vi "Actor Core.vi"(8 "error in":errorcluster, 11 "CameraTestingUI in":refnum<class "CameraTestingUI.lvclass">) -> (0 "error out":errorcluster, 3 "Actor out":refnum<class "Actor.lvclass">)   [LabVIEW 2020, in "CameraTestingUI.lvlib" / "CameraTestingUI.lvclass"]
doc: "(<B>Filename</B>: Actor Framework.lvlib:Actor.lvclass:Actor Core.vi)\n\nReceives messages to the actor, reacts to them, and initiates any error handling that may shut the actor down.\n\nDescendant classes may override this VI to append parallel tasks for the actor to complete while it handles messages. Overrides use the Call Parent Class Method node."
uses:
  CameraTestingUI.lvclass
  C:/Program Files (x86)/National Instruments/LabVIEW 2020/vi.lib/ActorFramework/Actor/Actor.lvclass
  <vilib>/ActorFramework/Actor/Actor.lvclass
  Private/TypeDef/ConnectCamera.ctl
  Private/TypeDef/DisconnectCamera.ctl
  Private/TypeDef/CommandParameters.ctl
  Private/TypeDef/SetParams.ctl
  Private/TypeDef/GetParams.ctl
  Private/TypeDef/SnapShot.ctl
  Private/TypeDef/StartStreamVideo.ctl
  Private/TypeDef/StopStreamVideo.ctl
  Private/TypeDef/Quit.ctl
  Private/TypeDef/ViewerTab.ctl
  Private/TypeDef/ConnectionStatus.ctl
  CameraTestingUI.lvclass/CameraTestingUI.ctl
  <vilib>/ActorFramework/Actor/Actor.lvclass/Actor.ctl
  <vilib>/ActorFramework/Message Enqueuer/Message Enqueuer.lvclass/Message Enqueuer.ctl
  Private/TypeDef/VideoLoopCamTestEvn.ctl
  ICameraTesting/ICameraTesting/TypeDef/VideoBufferUpdate.ctl
  <vilib>/picture/picture.llb/imagedata.ctl
  Private/TypeDef/HelperLoopCamTestEvn.ctl
  Camera/ICamera/ICamera/TypeDef/SnapInfo.ctl
  ICameraTesting/ICameraTesting/TypeDef/FrameRateValReceived.ctl
  ICameraTesting/ICameraTesting/TypeDef/ImgTypeValReceived.ctl
  ICameraTesting/ICameraTesting/TypeDef/ResolutionValReceived.ctl
  ICameraTesting/ICameraTesting/TypeDef/VideoOptCodesUpdated.ctl
  ICameraTesting/ICameraTesting/TypeDef/VideoOptionsInfo.ctl
  ICameraTesting/ICameraTesting/TypeDef/StatusUpdated.ctl
  ICameraTesting/ICameraTesting/TypeDef/StatusRecord.ctl
  CameraTestingUI Messages/onVideoOptInfoUpd Msg/onVideoOptInfoUpd Msg.lvclass/onVideoOptInfoUpd Msg.ctl
  CameraTestingUI Messages/onStatusUpdated Msg/onStatusUpdated Msg.lvclass/onStatusUpdated Msg.ctl
  ICameraTesting/ICameraTesting Messages/SetImageType Msg/SetImageType Msg.lvclass/SetImageType Msg.ctl
  ICameraTesting/ICameraTesting Messages/SetResolution Msg/SetResolution Msg.lvclass/SetResolution Msg.ctl
  ICameraTesting/ICameraTesting Messages/SetFrameRate Msg/SetFrameRate Msg.lvclass/SetFrameRate Msg.ctl
  <vilib>/ActorFramework/Message Enqueuer/Init from Existing Queue.vi
  <vilib>/ActorFramework/Message Enqueuer/Enqueue.vi
  CameraTestingUI Messages/onVideoOptInfoUpd Msg/onVideoOptInfoUpd Msg.lvclass
  C:/Program Files (x86)/National Instruments/LabVIEW 2020/vi.lib/ActorFramework/Message/Message.lvclass
  CameraTestingUI Messages/onStatusUpdated Msg/onStatusUpdated Msg.lvclass
  ICameraTesting/ICameraTesting Messages/ConnectCamera Msg/ConnectCamera Msg.lvclass
  ICameraTesting/ICameraTesting Messages/DisconnectCamera Msg/DisconnectCamera Msg.lvclass
  ICameraTesting/ICameraTesting Messages/SetImageType Msg/SetImageType Msg.lvclass
  ICameraTesting/ICameraTesting Messages/SetResolution Msg/SetResolution Msg.lvclass
  ICameraTesting/ICameraTesting Messages/SetFrameRate Msg/SetFrameRate Msg.lvclass
  ICameraTesting/ICameraTesting Messages/GetImageType Msg/GetImageType Msg.lvclass
  ICameraTesting/ICameraTesting Messages/GetResolution Msg/GetResolution Msg.lvclass
  ICameraTesting/ICameraTesting Messages/GetFrameRate Msg/GetFrameRate Msg.lvclass
  ICameraTesting/ICameraTesting Messages/SingleShot Msg/SingleShot Msg.lvclass
  ICameraTesting/ICameraTesting Messages/StartStreaming Msg/StartPlay Msg.lvclass
  ICameraTesting/ICameraTesting Messages/StopStreaming Msg/StopPlayMsg.lvclass
  <vilib>/ActorFramework/Stop Msg/Stop Msg.lvclass
  <vilib>/ActorFramework/Message Priority Queue/Priority Enqueue.vi
  <vilib>/ActorFramework/Message Enqueuer/Message Enqueuer.lvclass
  E:/GitHub/Evaluation_Test/Labview/src/CameraTestingApp/CameraTestingUI/CameraTestingUI/CameraTestingUI.lvclass
  E:/GitHub/Evaluation_Test/Labview/src/CameraTestingApp/ICameraTestingUI/ICameraTestingUI/ICameraTestingUI.lvclass
  ICameraTesting/ICameraTesting/ICameraTesting.lvclass
  Camera/ICamera/ICamera/ICamera.lvclass
panel:
  in  "ViewerTab":T1 caption="Viewer"
  out "ImgViewer":picture
  out "StatusLog":string caption="Status Log"
  in  "StopVideo":T2 caption="Stop"
  in  "PlayVideo":T3 caption="Play"
  in  "OneShot":T4 caption="SnapShot"
  in  "SetParam":T5 caption="Set Parameter"
  in  "GetParam":T6 caption="Get Paramameter"
  in  "CommParams":T7 caption="Command Parameters"
  out "ImgTypeInd":string caption="Last Value"
  in  "ImgTypeSlct":u8(ring) caption="List"
  out "ResolutionInd":string caption="Last Value"
  in  "ResSlct":u8(ring) caption="List"
  out "FrameRateInd":string caption="Last Value"
  in  "FrameRateSlct":u8(ring) caption="List"
  out "CameraLink":T8 caption="Connection status" items=["Disconnected", "Connected", "Error"]
  in  "Quit":T9
  in  "DisconnectCamera":T10 caption="Disconnect Camera"
  in  "ConnectCamera":T11 caption="Connect Camera"
  # "Parameters"
  # "Actions"
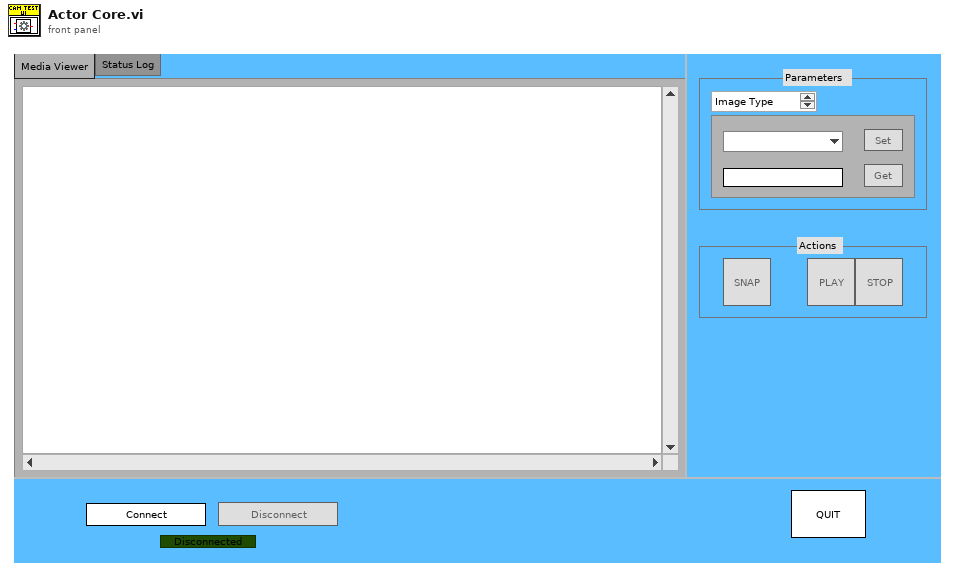
[diagram p1: front panel]
types:
  T1 = typedef "CameraTestingUI.lvlib/CameraTestingUI.lvclass/ViewerTab.ctl" = enum32{"Media Viewer", "Status Log"}
  T2 = typedef "CameraTestingUI.lvlib/CameraTestingUI.lvclass/StopStreamVideo.ctl" = bool
  T3 = typedef "CameraTestingUI.lvlib/CameraTestingUI.lvclass/StartStreamVideo.ctl" = bool
  T4 = typedef "CameraTestingUI.lvlib/CameraTestingUI.lvclass/SnapShot.ctl" = bool
  T5 = typedef "CameraTestingUI.lvlib/CameraTestingUI.lvclass/SetParams.ctl" = bool
  T6 = typedef "CameraTestingUI.lvlib/CameraTestingUI.lvclass/GetParams.ctl" = bool
  T7 = typedef "CameraTestingUI.lvlib/CameraTestingUI.lvclass/CommandParameters.ctl" = enum32{"Image Type", "Resolution", "Frame Rate"}
  T8 = typedef "CameraTestingUI.lvlib/CameraTestingUI.lvclass/ConnectionStatus.ctl" = u16
  T9 = typedef "CameraTestingUI.lvlib/CameraTestingUI.lvclass/Quit.ctl" = bool
  T10 = typedef "CameraTestingUI.lvlib/CameraTestingUI.lvclass/DisconnectCamera.ctl" = bool
  T11 = typedef "CameraTestingUI.lvlib/CameraTestingUI.lvclass/ConnectCamera.ctl" = bool
  T12 = typedef "CameraTestingUI.lvlib/CameraTestingUI.lvclass/HelperLoopEvntRegRef.ctl" = refnum<event-registration>
  T13 = typedef "CameraTestingUI.lvlib/CameraTestingUI.lvclass/VideoLoopEnvRgstRef.ctl" = refnum<event-registration>
  T14 = typedef "CameraTestingUI.lvlib/CameraTestingUI.lvclass/HelperLoopCamTestEvn.ctl" = cluster{"NewSnapData":refnum<user-event>, "FrameRateValReceived":T15, "ImgTypeValReceived":T16, "ResolutionValReceived":T17, "VideoOptInfoUpdated":T18, "StatusUpdated":T19}
  T15 = typedef "ICameraTesting.lvlib/ICameraTesting.lvclass/FrameRateValReceived.ctl" = refnum<user-event>
  T16 = typedef "ICameraTesting.lvlib/ICameraTesting.lvclass/ImgTypeValReceived.ctl" = refnum<user-event>
  T17 = typedef "ICameraTesting.lvlib/ICameraTesting.lvclass/ResolutionValReceived.ctl" = refnum<user-event>
  T18 = typedef "ICameraTesting.lvlib/ICameraTesting.lvclass/VideoOptCodesUpdated.ctl" = refnum<user-event>
  T19 = typedef "ICameraTesting.lvlib/ICameraTesting.lvclass/StatusUpdated.ctl" = refnum<user-event>
  T20 = typedef "imagedata.ctl" = cluster{"image type":i32, "image depth":i32, "image":u8[], "mask":u8[], "colors":u32[], "Rectangle":cluster{"left":i16, "top":i16, "right":i16, "bottom":i16}}
  T21 = typedef "ICameraTesting.lvlib/ICameraTesting.lvclass/VideoOptionsInfo.ctl" = cluster{"FrameRateCodesList":cluster{"Description":string, "Code":u8}[], "VideoResolutionCodesList":cluster{"Description":string, "Code":u8}[], "ImageTypeCodesList":cluster{"Description":string, "Code":u8}[]}
  T22 = typedef "ICameraTesting.lvlib/ICameraTesting.lvclass/StatusRecord.ctl" = cluster{"Time Stamp":timestamp, "Text":string, "Error":errorcluster}
  T23 = typedef "CameraTestingUI.lvlib/CameraTestingUI.lvclass/VideoLoopCamTestEvn.ctl" = cluster{"VideoBufferUpdate":T24}
  T24 = typedef "ICameraTesting.lvlib/ICameraTesting.lvclass/VideoBufferUpdate.ctl" = refnum<user-event>
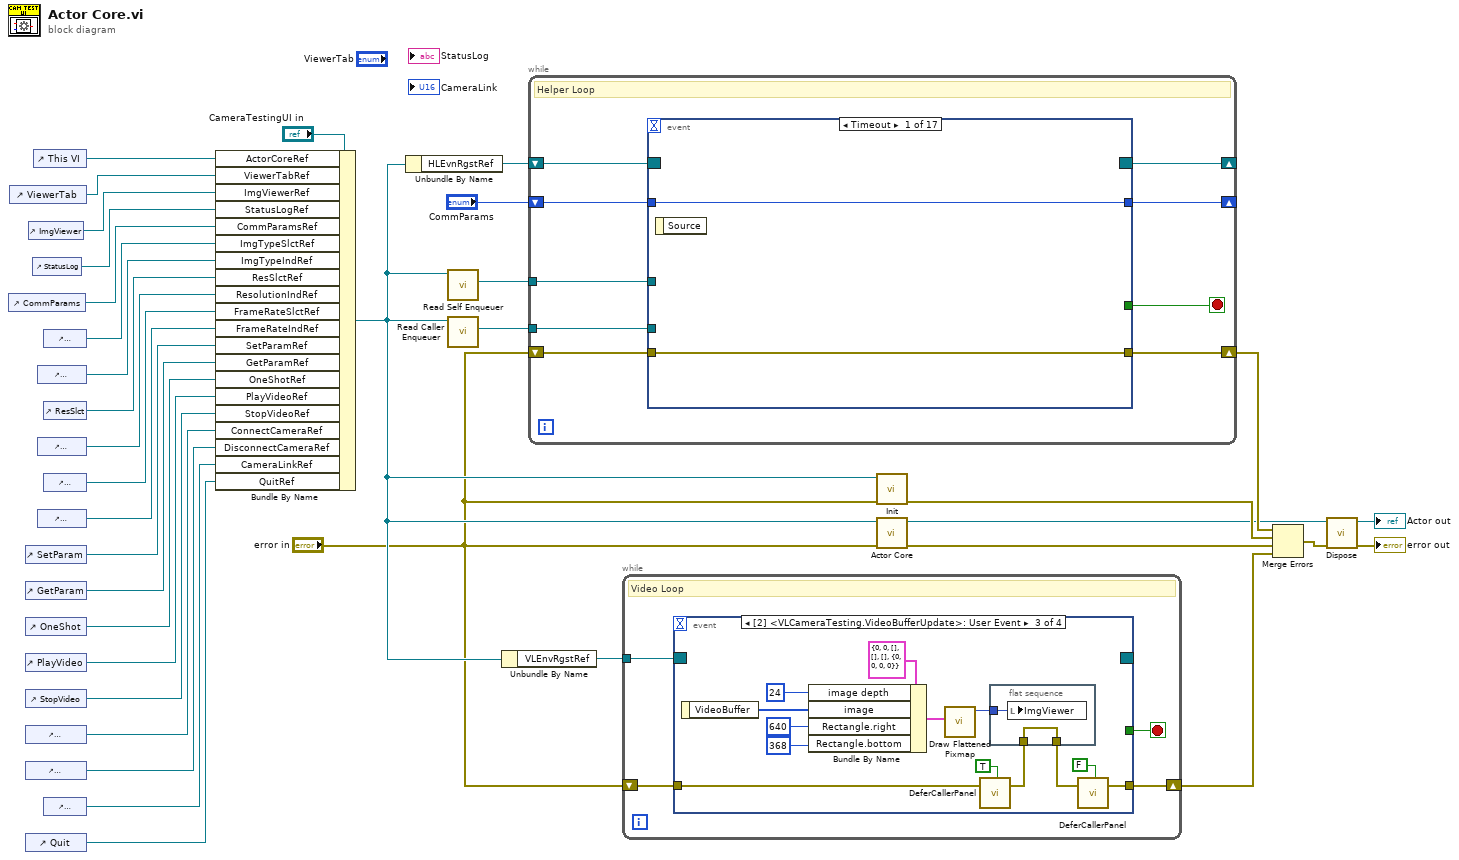
[diagram p0: block diagram]
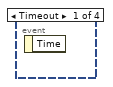
[diagram p2: hidden frame]
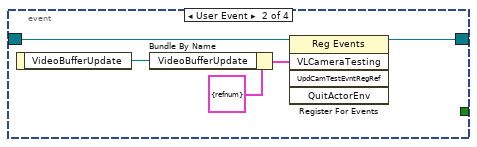
[diagram p3: hidden frame]
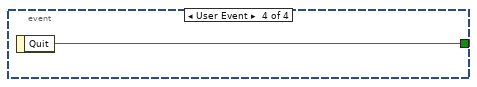
[diagram p4: hidden frame]
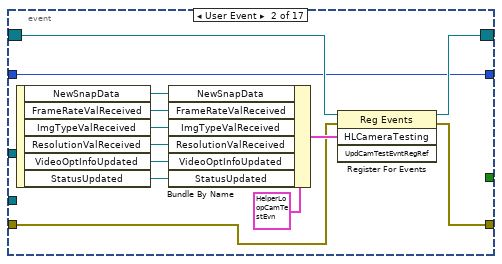
[diagram p5: hidden frame]
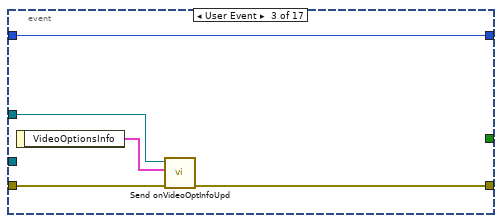
[diagram p6: hidden frame]
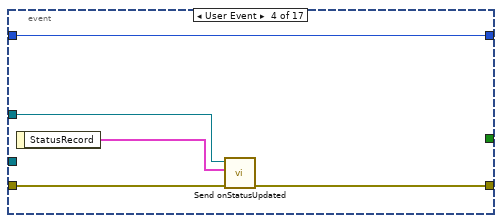
[diagram p7: hidden frame]
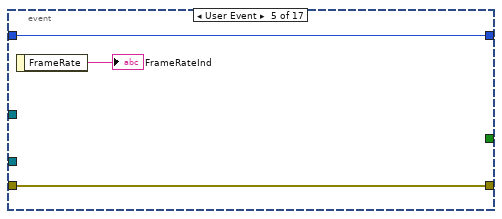
[diagram p8: hidden frame]
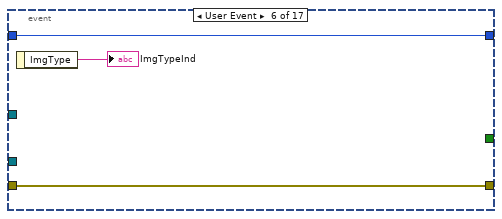
[diagram p9: hidden frame]
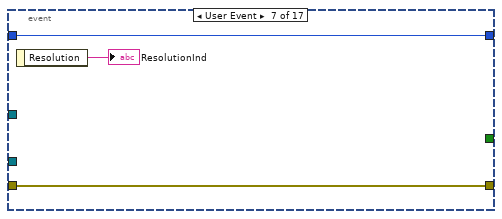
[diagram p10: hidden frame]
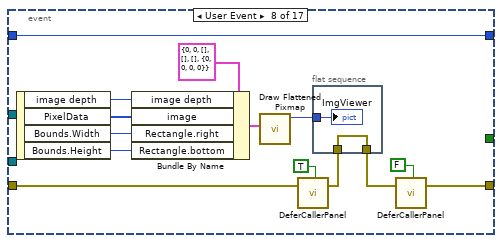
[diagram p11: hidden frame]
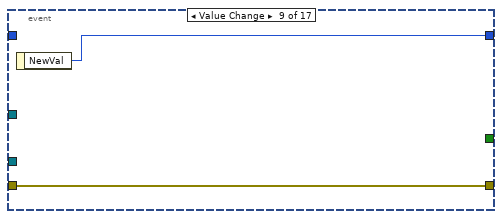
[diagram p12: hidden frame]
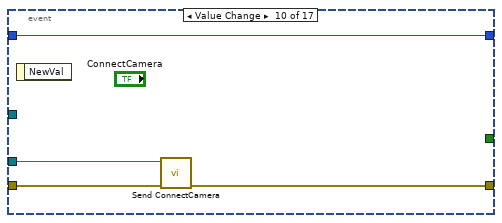
[diagram p13: hidden frame]
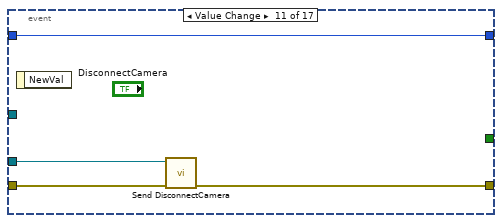
[diagram p14: hidden frame]
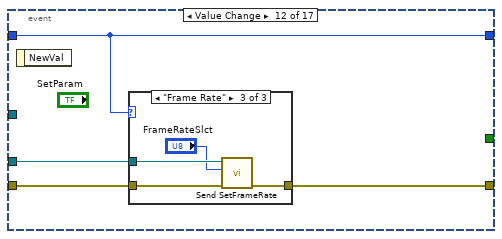
[diagram p15: hidden frame]
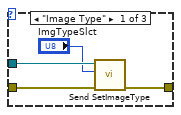
[diagram p16: hidden frame]
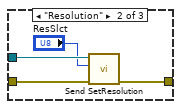
[diagram p17: hidden frame]
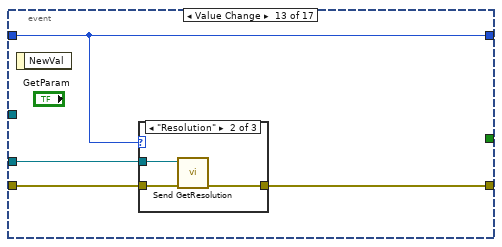
[diagram p18: hidden frame]
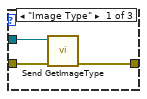
[diagram p19: hidden frame]
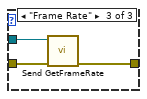
[diagram p20: hidden frame]
diagram:
  n1 = control-ref of="CommParams"() -> (w29:refnum<vi>)
  n2 = control-ref of="ViewerTab"() -> (w32:refnum<vi>)
  n3 = control-ref of="SetParam"() -> (w21:refnum<vi>)
  n4 = control-ref of="GetParam"() -> (w20:refnum<vi>)
  n5 = control-ref of="OneShot"() -> (w19:refnum<vi>)
  n6 = control-ref of="PlayVideo"() -> (w18:refnum<vi>)
  n7 = control-ref of="StopVideo"() -> (w17:refnum<vi>)
  n8 = control-ref of="ConnectCamera"() -> (w16:refnum<vi>)
  n9 = control-ref of="DisconnectCamera"() -> (w15:refnum<vi>)
  n10 = control-ref of="Quit"() -> (w11:refnum<vi>)
  n11 = control-ref of="ImgViewer"() -> (w31:refnum<vi>)
  n12 = control-ref of="StatusLog"() -> (w30:refnum<vi>)
  n13 = control-ref of="This VI"() -> (w34:refnum<vi>)
  n14 = control-ref of="ImgTypeInd"() -> (w27:refnum<vi>)
  n15 = control-ref of="ResolutionInd"() -> (w24:refnum<vi>)
  n16 = control-ref of="FrameRateInd"() -> (w22:refnum<vi>)
  n17 = control-ref of="ImgTypeSlct"() -> (w28:refnum<vi>)
  n18 = control-ref of="ResSlct"() -> (w25:refnum<vi>)
  n19 = control-ref of="FrameRateSlct"() -> (w23:refnum<vi>)
  n20 = control-ref of="CameraLink"() -> (w14:refnum<vi>)
  n21 = Bundle By Name(cluster="CameraTestingUI in", "ActorCoreRef"=w34, "ViewerTabRef"=w32, "ImgViewerRef"=w31, "StatusLogRef"=w30, "CommParamsRef"=w29, "ImgTypeSlctRef"=w28, "ImgTypeIndRef"=w27, "ResSlctRef"=w25, "ResolutionIndRef"=w24, "FrameRateSlctRef"=w23, "FrameRateIndRef"=w22, "SetParamRef"=w21, "GetParamRef"=w20, "OneShotRef"=w19, "PlayVideoRef"=w18, "StopVideoRef"=w17, "ConnectCameraRef"=w16, "DisconnectCameraRef"=w15, "CameraLinkRef"=w14, "QuitRef"=w11) -> (w12:refnum<class "CameraTestingUI.lvclass">)
  n22 = Unbundle By Name(w12) -> ("HLEvnRgstRef"=w33:T12)
  n23 = call <vilib>:"Read Self Enqueuer.vi"("Actor"=w12) -> ("Self Enqueuer"=w13:refnum<class "Message Enqueuer.lvclass">)  [unwired: 10 in]
  n24 = call <vilib>:"Read Caller Enqueuer.vi"("Actor"=w12) -> ("Caller Enqueuer"=w35:refnum<class "Message Enqueuer.lvclass">)  [unwired: 10 in]
  n25 = Unbundle By Name(w12) -> ("VLEnvRgstRef"=w10:T13)
  n26 = while {
    tunnel: w35 -> [w45]
    shift-right: [w43] -> _
    shift-left: "CommParams" -> [w44]
    shift-right: [w40] -> _
    shift-left: w33 -> [w41]
    tunnel: w13 -> [w39]
    shift-right: [w38] -> w8
    shift-left: "error in" -> [w37]
    stop <- w42 stop-if-true
    # "Helper Loop"
    n27 = event shown="[0] Timeout" {
      selector: w41 -> [_ w60 _ _ _ _ _ _ _ _ _ _ _ _ _ _ _]
      dyn-events: [_ w59 _ _ _ _ _ _ _ _ _ _ _ _ _ _ _] -> w40
      timeout: _ -> [_ _ _ _ _ _ _ _ _ _ _ _ _ _ _ _ _]
      tunnel: w45 -> [_ _ _ _ _ _ _ _ _ w101 w105 w109 w125 w137 w141 w145 w150]
      tunnel: w44 -> [w47 w58 w65 w68 w73 w75 w79 w93 _ w100 w104 w108 w124 w138 w142 w146 w152]
      tunnel: [w47 w58 w65 w68 w73 w75 w79 w93 w97 w100 w104 w108 w124 w138 w142 w146 w152] -> w43
      tunnel: w37 -> [w46 w49 w63 w70 w72 w74 w77 w85 w96 w99 w103 w107 w123 w136 w140 w144 w148]
      tunnel: [_ _ _ _ _ _ _ _ _ _ _ _ _ _ _ _ w151] -> w42
      tunnel: w39 -> [_ _ w64 w66 _ _ _ _ _ _ _ _ _ _ _ _ _]
      tunnel: [w46 w48 w61 w69 w72 w74 w77 w82 w96 w98 w102 w106 w122 w135 w139 w143 w147] -> w38
      event Timeout {
        n28 = event-data() -> ()  [unwired: 1 in, 1 out]
      }
      event User Event {
        n29 = event-data() -> ("NewSnapData"=w57:refnum<user-event>, "FrameRateValReceived"=w56:T15, "ImgTypeValReceived"=w55:T16, "ResolutionValReceived"=w54:T17, "VideoOptInfoUpdated"=w53:T18, "StatusUpdated"=w52:T19)  [unwired: 1 in]
        n30 = Bundle By Name(cluster=T14 {"NewSnapData"=refnum, "FrameRateValReceived"=refnum, "ImgTypeValReceived"=refnum, "ResolutionValReceived"=refnum, "VideoOptInfoUpdated"=refnum, "StatusUpdated"=refnum} ("HelperLoopEvn"), "NewSnapData"=w57, "FrameRateValReceived"=w56, "ImgTypeValReceived"=w55, "ResolutionValReceived"=w54, "VideoOptInfoUpdated"=w53, "StatusUpdated"=w52) -> (w50:T14)
        n31 = register-events(reference=w60, error in=w49, w50) -> (reference out=w59:T12, error out=w48:errorcluster)  [unwired: 1 in]
      }
      event User Event {
        n32 = event-data() -> ("VideoOptionsInfo"=w62:T21)  [unwired: 1 in]
        n33 = call "Send onVideoOptInfoUpd.vi"("error in (no error)"=w63, "VideoOptionsInfo"=w62, "Message Enqueuer"=w64) -> ("error out"=w61:errorcluster)  [unwired: 7 in, 1 out]
      }
      event User Event {
        n34 = event-data() -> ("StatusRecord"=w67:T22)  [unwired: 1 in]
        n35 = call "Send onStatusUpdated.vi"("error in (no error)"=w70, "StatusRecord"=w67, "Message Enqueuer"=w66) -> ("error out"=w69:errorcluster)  [unwired: 7 in, 1 out]
      }
      event User Event {
        n36 = event-data() -> ("FrameRate"=→"FrameRateInd":string)  [unwired: 1 in]
      }
      event User Event {
        n37 = event-data() -> ("ImgType"=→"ImgTypeInd":string)  [unwired: 1 in]
      }
      event User Event {
        n38 = event-data() -> ("Resolution"=→"ResolutionInd":string)  [unwired: 1 in]
      }
      event User Event {
        n39 = event-data() -> ("image depth"=w91:i32, "PixelData"=w90:u8[], "Bounds.Width"=w89:i16, "Bounds.Height"=w88:i16)  [unwired: 1 in]
        n40 = Bundle By Name(cluster=T20 {"image type"=0, "image depth"=0, "image"=[], "mask"=[], "colors"=[], "Rectangle"={"left"=0, "top"=0, "right"=0, "bottom"=0}} ("image data"), "image depth"=w91, "image"=w90, "Rectangle.right"=w89, "Rectangle.bottom"=w88) -> (w87:T20)
        n41 = call <vilib>:"Draw Flattened Pixmap.vi"("image data"=w87) -> ("new picture"=w86:picture)  [unwired: 8 in]
        n42 = call "DeferCallerPanel.vi"("On/Off"=TRUE, "error in (no error)"=w85) -> ("error out"=w84:errorcluster)  [unwired: 17 in]
        n43 = flat-sequence {
          tunnel: w86 -> [w95]
          tunnel: w84 -> [w94]
          tunnel: [w94] -> w83
          frame #0 {
            "ImgViewer" <- w95
          }
        }
        n44 = call "DeferCallerPanel.vi"("On/Off"=FALSE, "error in (no error)"=w83) -> ("error out"=w82:errorcluster)  [unwired: 17 in]
      }
      event Value Change {
        n45 = event-data() -> ("NewVal"=w97:T7)  [unwired: 1 in]
      }
      event Value Change {
        n46 = event-data() -> ()  [unwired: 1 in, 1 out]
        n47 = call "Send ConnectCamera.vi"("error in (no error)"=w99, "Message Enqueuer"=w101) -> ("error out"=w98:errorcluster)  [unwired: 8 in, 1 out]
      }
      event Value Change {
        n48 = event-data() -> ()  [unwired: 1 in, 1 out]
        n49 = call "Send DisconnectCamera.vi"("error in (no error)"=w103, "Message Enqueuer"=w105) -> ("error out"=w102:errorcluster)  [unwired: 8 in, 1 out]
      }
      event Value Change {
        n50 = event-data() -> ()  [unwired: 1 in, 1 out]
        n51 = case shown="\"Frame Rate\"" w108 {
          tunnel: w109 -> [w113 w117 w121]
          tunnel: w107 -> [w111 w115 w119]
          tunnel: [w110 w114 w118] -> w106
          frame "Image Type" {
            n52 = call "Send SetImageType.vi"("error in (no error)"=w111, "Image Type"="ImgTypeSlct", "Message Enqueuer"=w113) -> ("error out"=w110:errorcluster)  [unwired: 7 in, 1 out]
          }
          frame "Resolution" {
            n53 = call "Send SetResolution.vi"("error in (no error)"=w115, "Resolution"="ResSlct", "Message Enqueuer"=w117) -> ("error out"=w114:errorcluster)  [unwired: 7 in, 1 out]
          }
          frame "Frame Rate" {
            n54 = call "Send SetFrameRate.vi"("error in (no error)"=w119, "Frame Rate"="FrameRateSlct", "Message Enqueuer"=w121) -> ("error out"=w118:errorcluster)  [unwired: 7 in, 1 out]
          }
        }
      }
      event Value Change {
        n55 = event-data() -> ()  [unwired: 1 in, 1 out]
        n56 = case shown="\"Resolution\"" w124 {
          tunnel: w125 -> [w128 w131 w134]
          tunnel: w123 -> [w127 w130 w133]
          tunnel: [w126 w129 w132] -> w122
          frame "Image Type" {
            n57 = call "Send GetImageType.vi"("error in (no error)"=w127, "Message Enqueuer"=w128) -> ("error out"=w126:errorcluster)  [unwired: 8 in, 1 out]
          }
          frame "Resolution" {
            n58 = call "Send GetResolution.vi"("error in (no error)"=w130, "Message Enqueuer"=w131) -> ("error out"=w129:errorcluster)  [unwired: 8 in, 1 out]
          }
          frame "Frame Rate" {
            n59 = call "Send GetFrameRate.vi"("error in (no error)"=w133, "Message Enqueuer"=w134) -> ("error out"=w132:errorcluster)  [unwired: 8 in, 1 out]
          }
        }
      }
      event Value Change {
        n60 = event-data() -> ()  [unwired: 1 in, 1 out]
        n61 = call "Send SingleShot.vi"("error in (no error)"=w136, "Message Enqueuer"=w137) -> ("error out"=w135:errorcluster)  [unwired: 8 in, 1 out]
      }
      event Value Change {
        n62 = event-data() -> ()  [unwired: 1 in, 1 out]
        n63 = call "Send StartPlay.vi"("error in (no error)"=w140, "Message Enqueuer"=w141) -> ("error out"=w139:errorcluster)  [unwired: 8 in, 1 out]
      }
      event Value Change {
        n64 = event-data() -> ()  [unwired: 1 in, 1 out]
        n65 = call "Send StopPlay.vi"("error in (no error)"=w144, "Message Enqueuer"=w145) -> ("error out"=w143:errorcluster)  [unwired: 8 in, 1 out]
      }
      event Value Change {
        n66 = event-data() -> ("NewVal"=w151:T9)  [unwired: 1 in]
        n67 = call <vilib>:"Send Normal Stop.vi"("Message Enqueuer"=w150) -> ("error out"=w149:errorcluster)  [unwired: 10 in]
        n68 = Merge Errors(w148, w149) -> (w147:errorcluster)
      }
    }
  }
  n69 = while {
    tunnel: w10 -> [w156]
    shift-right: [w153] -> w1
    shift-left: "error in" -> [w154]
    stop <- w155 stop-if-true
    # "Video Loop"
    n70 = event shown="[2] <VLCameraTesting.VideoBufferUpdate>: User Event" {
      selector: w156 -> [_ w161 _ _]
      dyn-events: [_ w160 _ _] -> _
      timeout: _ -> [_ _ _ _]
      tunnel: [_ _ _ w177] -> w155
      tunnel: w154 -> [_ _ w165 _]
      tunnel: [_ _ w164 _] -> w153
      event Timeout {
        n71 = event-data() -> ()  [unwired: 1 in, 1 out]
      }
      event User Event {
        n72 = event-data() -> ("VideoBufferUpdate"=w159:T24)  [unwired: 1 in]
        n73 = Bundle By Name(cluster=T23 {"VideoBufferUpdate"=refnum} ("event source"), "VideoBufferUpdate"=w159) -> (w158:T23)
        n74 = register-events(reference=w161, w158) -> (reference out=w160:T13)  [unwired: 3 in, 1 out]
      }
      event User Event {
        n75 = event-data() -> ("VideoBuffer"=w168:u8[])  [unwired: 1 in]
        n76 = Bundle By Name(cluster=T20 {"image type"=0, "image depth"=0, "image"=[], "mask"=[], "colors"=[], "Rectangle"={"left"=0, "top"=0, "right"=0, "bottom"=0}} ("image data"), "image depth"=24, "image"=w168, "Rectangle.right"=i16 640, "Rectangle.bottom"=i16 368) -> (w170:T20)
        n77 = call <vilib>:"Draw Flattened Pixmap.vi"("image data"=w170) -> ("new picture"=w169:picture)  [unwired: 8 in]
        n78 = call "DeferCallerPanel.vi"("On/Off"=TRUE, "error in (no error)"=w165) -> ("error out"=w167:errorcluster)  [unwired: 17 in]
        n79 = flat-sequence {
          tunnel: w169 -> [w176]
          tunnel: [w175] -> w166
          tunnel: w167 -> [w175]
          frame #0 {
            n80 = local write "ImgViewer"(w176) -> ()
          }
        }
        n81 = call "DeferCallerPanel.vi"("On/Off"=FALSE, "error in (no error)"=w166) -> ("error out"=w164:errorcluster)  [unwired: 17 in]
      }
      event User Event {
        n82 = event-data() -> ("Quit"=w177:bool)  [unwired: 1 in]
      }
    }
  }
  n83 = call "Init.vi"("error in (no error)"="error in", "CameraTestingUI in"=w12) -> ("error out"=w7:errorcluster)  [unwired: 8 in, 1 out]
  n84 = call-parent "Actor Core.vi"("error in"="error in", "Actor in"=w12) -> ("error out"=w6:errorcluster, "Actor out"=w2:refnum<class "Actor.lvclass">)  [unwired: 8 in]
  n85 = Merge Errors(w8, w7, w6, w1) -> (w3:errorcluster)
  n86 = call "Dispose.vi"("error in (no error)"=w3, "Actor in"=w2) -> ("error out"=→"error out":errorcluster, "Actor out"=→"Actor out":refnum<class "Actor.lvclass">)  [unwired: 8 in]
